vi "TS Register Event Callbacks.vi"(8 "error in (no error)":errorcluster, 11 "Auto UI in":refnum<class "Auto UI.lvclass">) -> (0 "error out":errorcluster, 3 "Auto UI out":refnum<class "Auto UI.lvclass">)   [LabVIEW 2023, in "GUI.lvlib" / "Auto UI.lvlib" / "Auto UI.lvclass"]
uses:
  Auto UI.lvclass
  Auto UI.lvclass/Auto UI.ctl
  TS Event Callback/DisplayExecution Event Callback.vi
  TS Event Callback/DisplaySequenceFile Event Callback.vi
  TS Event Callback/ExitApplication Event Callback.vi
  TS Event Callback/ReportError Event Callback.vi
  TS Event Callback/Wait Event Callback.vi
  TS Event Callback/User Message Teststand Event Callback.vi
  TS Event Callback/UI Message Teststand Event Callback.vi
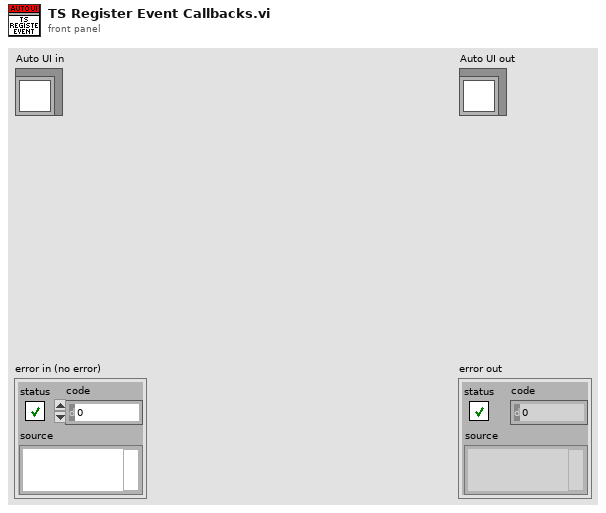
[diagram p1: front panel]
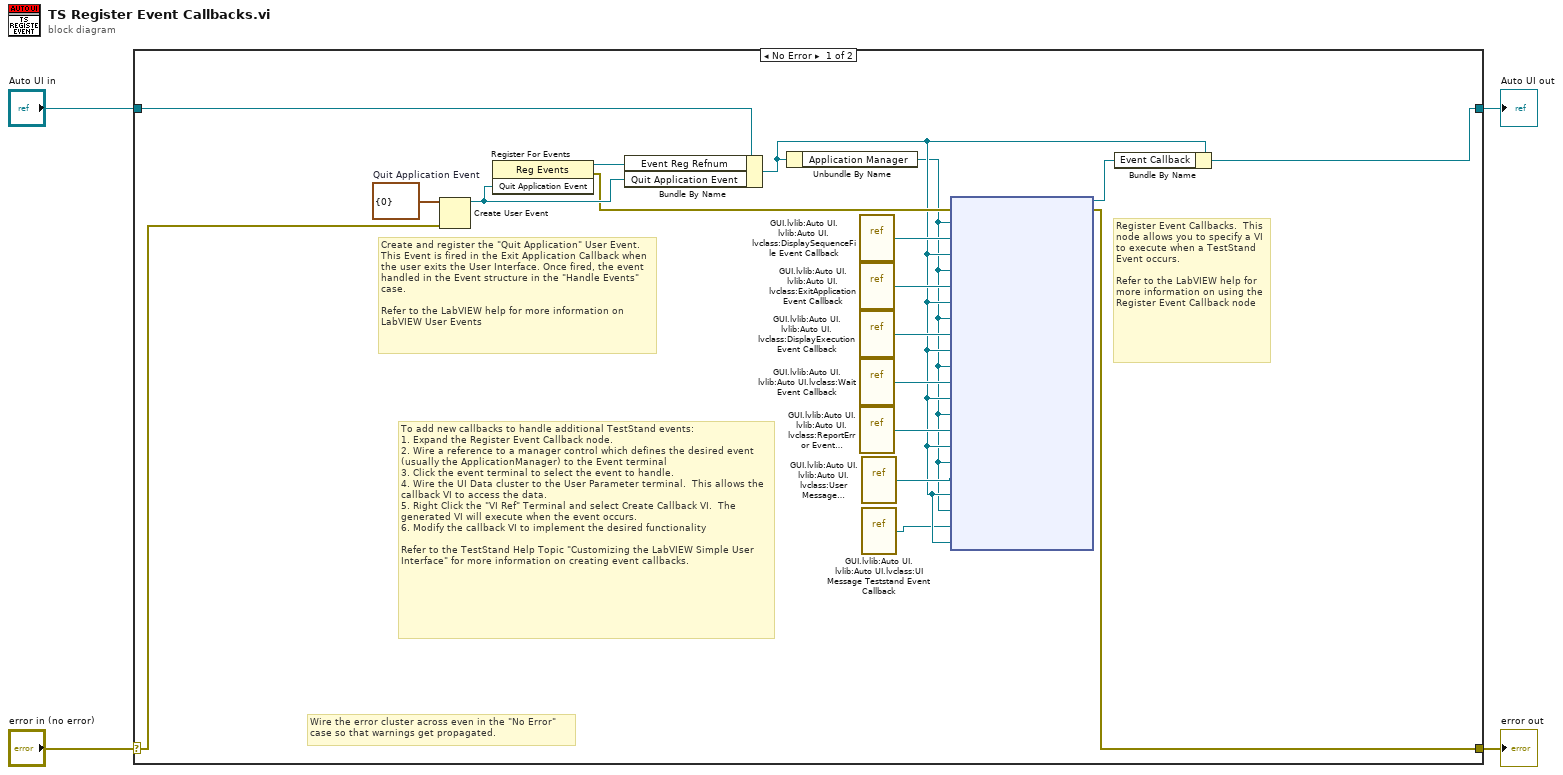
[diagram p0: block diagram]
diagram:
  n1 = case shown="No Error" "error in (no error)" {
    selector: "error in (no error)" -> [w16 w24]
    tunnel: [w14 w24] -> w3
    tunnel: [w15 w23] -> w1
    tunnel: "Auto UI in" -> [w17 w23]
    frame No Error {
      w22 = cluster{"Number":i32} {"Number"=0}  # Quit Application Event
      # "Register Event Callbacks.  This node allows you to specify a VI to execute when a TestStand Event occurs. \n\nRefer to the LabVIEW help for more information on using the Register Event Callback node"
      # "Create and register the \"Quit Application\" User Event. This Event is fired in the Exit Application Callback when the user exits the User Interface. Once fired, the event handled in the Event structure in the \"Handle Events\" case.\n\nRefer to the LabVIEW help for more information on LabVIEW User Events"
      # "To add new callbacks to handle additional TestStand events:\n1. Expand the Register Event Callback node.  \n2. Wire a reference to a manager control which defines the desired event (usually the ApplicationManager) to the Event terminal\n3. Click the event terminal to select the event to handle.\n4. Wire the UI Data cluster to the User Parameter terminal.  This allows the callback VI to access the data.\n5. Right Click the \"VI Ref\" Terminal and select Create Callback VI.  The generated VI will execute when the event occurs.\n6. Modify the callback VI to implement the desired functionality\n\nRefer to the TestStand Help Topic \"Customizing the LabVIEW Simple User Interface\" for more information on creating event callbacks."
      # "Wire the error cluster across even in the \"No Error\"\ncase so that warnings get propagated."
      n2 = Create User Event(user event datatype=w22, error in=w16) -> (user event=w20:refnum<user-event>)  [unwired: 1 out]
      n3 = register-events(w20) -> (reference out=w19:refnum<event-registration>, error out=w18:errorcluster)  [unwired: 2 in]
      n4 = Bundle By Name(cluster=w17, "Event Reg Refnum"=w19, "Quit Application Event"=w20) -> (w7:refnum<class "Auto UI.lvclass">)
      n5 = Unbundle By Name(w7) -> ("Application Manager"=w5:refnum<k7>)
      n6 = vi-ref "GUI.lvlib:Auto UI.lvlib:Auto UI.lvclass:DisplaySequenceFile Event Callback.vi"() -> (w12:refnum<vi>)
      n7 = vi-ref "GUI.lvlib:Auto UI.lvlib:Auto UI.lvclass:ExitApplication Event Callback.vi"() -> (w13:refnum<vi>)
      n8 = vi-ref "GUI.lvlib:Auto UI.lvlib:Auto UI.lvclass:DisplayExecution Event Callback.vi"() -> (w11:refnum<vi>)
      n9 = vi-ref "GUI.lvlib:Auto UI.lvlib:Auto UI.lvclass:Wait Event Callback.vi"() -> (w10:refnum<vi>)
      n10 = vi-ref "GUI.lvlib:Auto UI.lvlib:Auto UI.lvclass:ReportError Event Callback.vi"() -> (w9:refnum<vi>)
      n11 = vi-ref "GUI.lvlib:Auto UI.lvlib:Auto UI.lvclass:User Message Teststand Event Callback.vi"() -> (w8:refnum<vi>)
      n12 = vi-ref "GUI.lvlib:Auto UI.lvlib:Auto UI.lvclass:UI Message Teststand Event Callback.vi"() -> (w6:refnum<vi>)
      n13 = node(w18, w5, w12, w7, w5, w13, w7, w5, w11, w7, w5, w10, w7, w5, w9, w7, w5, w8, w7, w5, w6, w7) -> (w21:refnum<k27>, w14:errorcluster)  [unwired: 1 in]
      n14 = Bundle By Name(cluster=w7, "Event Callback"=w21) -> (w15:refnum<class "Auto UI.lvclass">)
    }
    frame Error {
    }
  }
  "error out" <- w3
  "Auto UI out" <- w1
